vi "SDI Init SDI.vi"(9 "SDIIndex":u8, 10 "DevIndex":i32, 11 "DevType":i32) -> (3 "function return":i32)   [LabVIEW 2010, in "ControlSDI.lvlib"]
doc: "int WINAPI SDI_InitSDI(int DevType, int DevIndex, unsigned char SDIIndex);"
uses:
  ControlSDI.lvlib
  ControlSDI/Ginkgo_Driver.dll
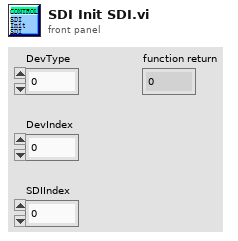
[diagram p1: front panel]
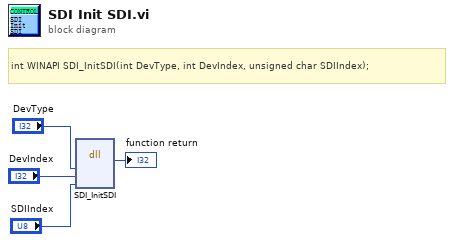
[diagram p0: block diagram]
diagram:
  # "int WINAPI SDI_InitSDI(int DevType, int DevIndex, unsigned char SDIIndex);"
  n1 = dll-call lib="E:/Project/vt_ginkgo/truck/Ginkgo Driver/vs2010/Ginkgo_USB-I2C&SPI&CAN_API_v2.0.3.3/lib/labview_32bit/ControlSDI/Ginkgo_Driver.*" fn="SDI_InitSDI"("DevType"="DevType", "DevIndex"="DevIndex", "SDIIndex"="SDIIndex") -> (→"function return":i32)  [unwired: 6 in, 2 out]
